vi "General_Setup_string.vi"() -> (0 "Output string":string)   [LabVIEW 2017]
uses:
  Controls/Graph_Type.ctl
  Globals/Preference_global.vi
  Globals/Meas_global.vi
  Globals/Trav_pos_global.vi
panel:
  in  "Plot Type":T1=enum."Voltage trace"
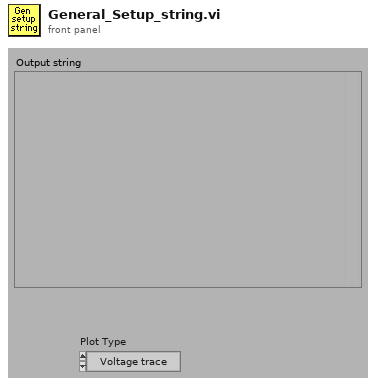
[diagram p1: front panel]
types:
  T1 = typedef "Graph_Type.ctl" = enum16{"Show no graph", "Voltage trace", "Velocity trace", "Vel histogram", "Spectrum", "f.E(f) v Log f", "Auto-Corr"}
  T2 = enum16{"From String to Cluster", "From Cluster to String"}
  T3 = cluster{"Plot 1":u16, "Plot 2":u16, "Save graph":u16, "Plot Type":T1}
  T4 = enum16{"Save no data", "Save data in new files", "Save data in existing files"}
  T5 = typedef "Tunnel_Coordinates.ctl" = enum16{"Work in Tunnel Coordinates", "Work in Model Coordinates"}
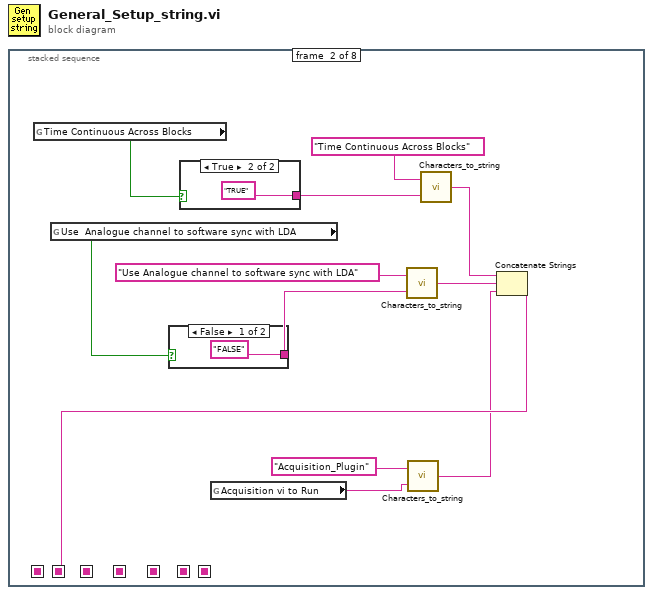
[diagram p0: block diagram]
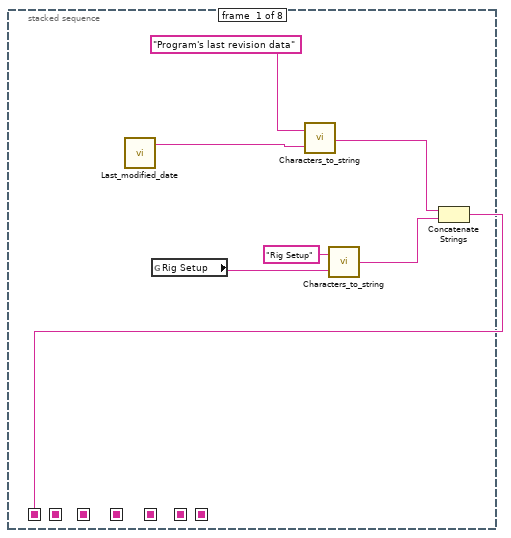
[diagram p2: hidden frame]
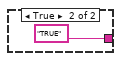
[diagram p3: hidden frame]
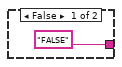
[diagram p4: hidden frame]
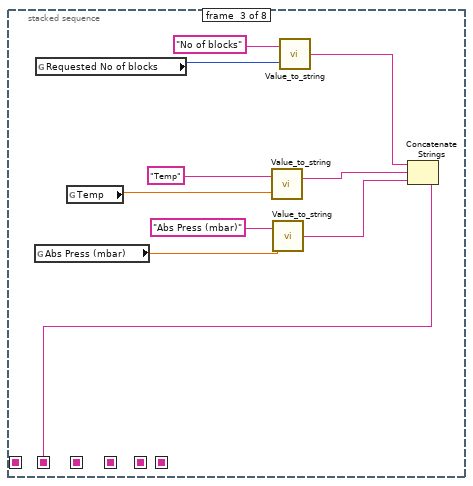
[diagram p5: hidden frame]
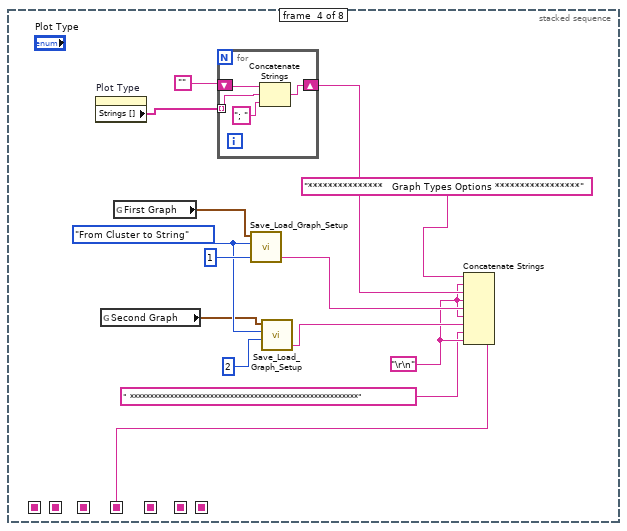
[diagram p6: hidden frame]
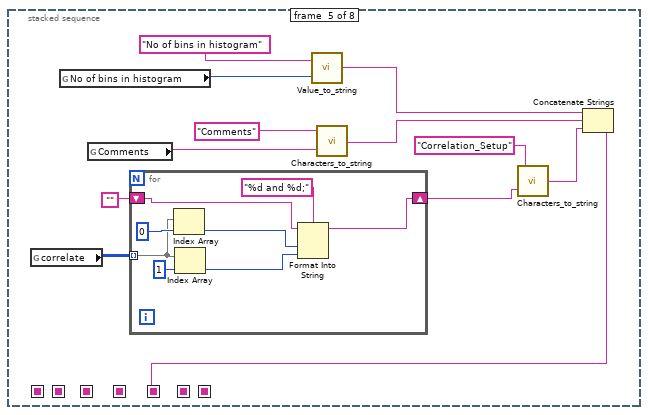
[diagram p7: hidden frame]
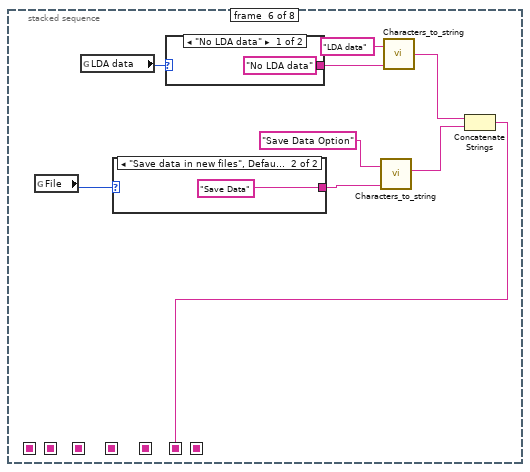
[diagram p8: hidden frame]
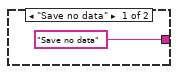
[diagram p9: hidden frame]
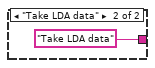
[diagram p10: hidden frame]
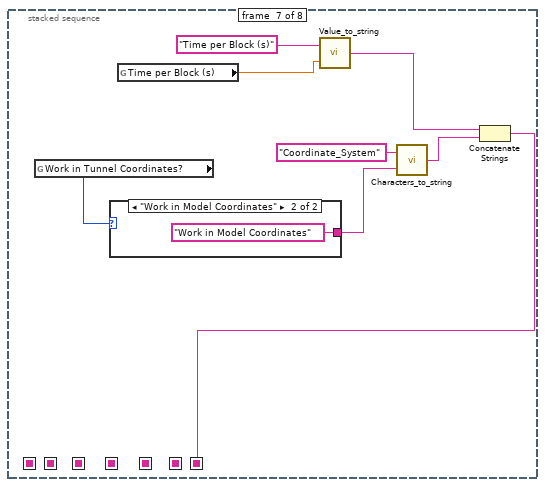
[diagram p11: hidden frame]
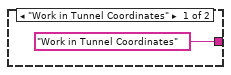
[diagram p12: hidden frame]
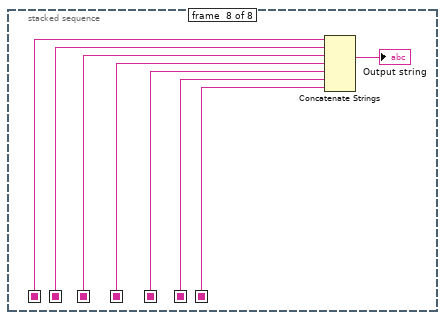
[diagram p13: hidden frame]
diagram:
  n1 = stacked-sequence {
    seq-local: [_ _ w31 _ _ _ _ _] -> [_ _ _ _ _ _ _ w102]
    seq-local: [_ w15 _ _ _ _ _ _] -> [_ _ _ _ _ _ _ w101]
    seq-local: [_ _ _ _ _ w72 _ _] -> [_ _ _ _ _ _ _ w97]
    seq-local: [_ _ _ _ _ _ w92 _] -> [_ _ _ _ _ _ _ w96]
    seq-local: [_ _ _ w47 _ _ _ _] -> [_ _ _ _ _ _ _ w99]
    seq-local: [_ _ _ _ w58 _ _ _] -> [_ _ _ _ _ _ _ w98]
    seq-local: [w7 _ _ _ _ _ _ _] -> [_ _ _ _ _ _ _ w95]
    frame #0 {
      n2 = call "Last_modified_date.vi"() -> ("RevisionString"=w2:string)  [unwired: 1 in, 1 out]
      n3 = global read "Preference_global.vi" "Rig Setup"() -> (w4:string)
      n4 = call "Characters_to_string.vi"("Characters to write"=w2, "Label for characters"="Program's last revision data") -> ("Output string"=w1:string)
      n5 = call "Characters_to_string.vi"("Characters to write"=w4, "Label for characters"="Rig Setup") -> ("Output string"=w5:string)
      n6 = Concatenate Strings(w1, w5) -> (w7:string)
    }
    frame #1 {
      n7 = global read "Meas_global.vi" "Time Continuous Across Blocks"() -> (w14:bool)
      n8 = global read "Meas_global.vi" "Use  Analogue channel to software sync with LDA"() -> (w12:bool)
      n9 = case shown="False" w12 {
        tunnel: ["FALSE" "TRUE"] -> w11
        frame False {
        }
        frame True {
        }
      }
      n10 = case shown="True" w14 {
        tunnel: ["FALSE" "TRUE"] -> w13
        frame False {
        }
        frame True {
        }
      }
      n11 = global read "Meas_global.vi" "Acquisition vi to Run"() -> (w8:string)
      n12 = call "Characters_to_string.vi"("Characters to write"=w11, "Label for characters"="Use Analogue channel to software sync with LDA") -> ("Output string"=w16:string)
      n13 = call "Characters_to_string.vi"("Characters to write"=w8, "Label for characters"="Acquisition_Plugin") -> ("Output string"=w9:string)
      n14 = call "Characters_to_string.vi"("Characters to write"=w13, "Label for characters"="Time Continuous Across Blocks") -> ("Output string"=w17:string)
      n15 = Concatenate Strings(w17, w16, w9) -> (w15:string)
    }
    frame #2 {
      n16 = global read "Meas_global.vi" "Abs Press (mbar)"() -> (w28:dbl)
      n17 = global read "Meas_global.vi" "Requested No of blocks"() -> (w32:i32)
      n18 = global read "Meas_global.vi" "Temp"() -> (w27:dbl)
      n19 = call "Value_to_string.vi"("Value"=w27, "Label for value"="Temp") -> ("Output string"=w26:string)  [unwired: 1 in]
      n20 = call "Value_to_string.vi"("Value"=w28, "Label for value"="Abs Press (mbar)") -> ("Output string"=w25:string)  [unwired: 1 in]
      n21 = call "Value_to_string.vi"("Value"=w32, "Label for value"="No of blocks") -> ("Output string"=w24:string)  [unwired: 1 in]
      n22 = Concatenate Strings(w24, w26, w25) -> (w31:string)
    }
    frame #3 {
      w37 = "\r\n"
      w44 = T2."From Cluster to String" ("Mode")
      n23 = property on="Plot Type" class="Enum (strict)"() -> ("Strings []"=w39:string[])  [unwired: 2 in, 2 out]
      n24 = global read "Meas_global.vi" "Second Graph"() -> (w43:T3)
      n25 = global read "Meas_global.vi" "First Graph"() -> (w40:T3)
      n26 = for {
        shift-right: [w50] -> w38
        shift-left: "" -> [w51]
        tunnel: w39 -> [w49] mode=indexing
        n27 = Concatenate Strings(w51, w49, "; " ("string")) -> (w50:string)
      }
      n28 = call "Save_Load_Graph_Setup.vi"("Graph Number"=1, "Mode"=w44, "Graph in"=w40) -> ("Setup String Out"=w41:string)  [unwired: 1 in, 2 out]
      n29 = call "Save_Load_Graph_Setup.vi"("Graph Number"=2, "Mode"=w44, "Graph in"=w43) -> ("Setup String Out"=w42:string)  [unwired: 1 in, 2 out]
      n30 = Concatenate Strings("***************   Graph Types Options *****************", w37, w38, w37, w41, w37, w42, " *********************************************************" ("string"), w37) -> (w47:string)
    }
    frame #4 {
      n31 = global read "Meas_global.vi" "correlate"() -> (w56:i32[][])
      n32 = global read "Meas_global.vi" "No of bins in histogram"() -> (w62:i32)
      n33 = global read "Meas_global.vi" "Comments"() -> (w57:string)
      n34 = for {
        tunnel: w56 -> [w69] mode=indexing
        shift-right: [w65] -> w53
        shift-left: "" -> [w66]
        n35 = Index Array(array=w69, index=0) -> (element=w68:i32)
        n36 = Index Array(array=w69, index=1) -> (element=w67:i32)
        n37 = Format Into String(format string="%d and %d;", initial string=w66, w68, w67) -> (resulting string=w65:string)  [unwired: 1 in, 1 out]
      }
      n38 = call "Value_to_string.vi"("Value"=w62, "Label for value"="No of bins in histogram") -> ("Output string"=w61:string)  [unwired: 1 in]
      n39 = call "Characters_to_string.vi"("Characters to write"=w57, "Label for characters"="Comments") -> ("Output string"=w59:string)
      n40 = call "Characters_to_string.vi"("Characters to write"=w53, "Label for characters"="Correlation_Setup") -> ("Output string"=w52:string)
      n41 = Concatenate Strings(w61, w59, w52) -> (w58:string)
    }
    frame #5 {
      n42 = global read "Meas_global.vi" "File"() -> (w77:T4)
      n43 = global read "Meas_global.vi" "LDA data"() -> (w78:enum16{"No LDA data", "Take LDA data"})
      n44 = case shown="\"Save data in new files\", Default" w77 {
        tunnel: ["Save no data" "Save Data"] -> w75
        frame "Save no data" {
        }
        frame "Save data in new files", Default {
        }
      }
      n45 = case shown="\"No LDA data\"" w78 {
        tunnel: ["No LDA data" "Take LDA data"] -> w79
        frame "No LDA data" {
        }
        frame "Take LDA data" {
        }
      }
      n46 = call "Characters_to_string.vi"("Characters to write"=w75, "Label for characters"="Save Data Option") -> ("Output string"=w73:string)
      n47 = call "Characters_to_string.vi"("Characters to write"=w79, "Label for characters"="LDA data") -> ("Output string"=w74:string)
      n48 = Concatenate Strings(w74, w73) -> (w72:string)
    }
    frame #6 {
      n49 = global read "Trav_pos_global.vi" "Work in Tunnel Coordinates?"() -> (w91:T5)
      n50 = case shown="\"Work in Model Coordinates\"" w91 {
        tunnel: ["Work in Tunnel Coordinates" "Work in Model Coordinates"] -> w90
        frame "Work in Tunnel Coordinates" {
        }
        frame "Work in Model Coordinates" {
        }
      }
      n51 = global read "Meas_global.vi" "Time per Block (s)"() -> (w85:dbl)
      n52 = call "Value_to_string.vi"("Value"=w85, "Label for value"="Time per Block (s)") -> ("Output string"=w86:string)  [unwired: 1 in]
      n53 = call "Characters_to_string.vi"("Characters to write"=w90, "Label for characters"="Coordinate_System") -> ("Output string"=w88:string)
      n54 = Concatenate Strings(w86, w88) -> (w92:string)
    }
    frame #7 {
      n55 = Concatenate Strings(w95, w101, w102, w99, w98, w97, w96) -> (→"Output string":string)
    }
  }
